vi "HELP.vi"(8 "error in (no error)":errorcluster, 11 "Instrument in":refnum<class "Instrument.lvclass">) -> (0 "error out":errorcluster, 2 "Commands":string[](array[string]), 3 "Instrument out":refnum<class "Instrument.lvclass">)   [LabVIEW 2016, in "Instrument.lvclass"]
uses:
  Instrument.lvclass
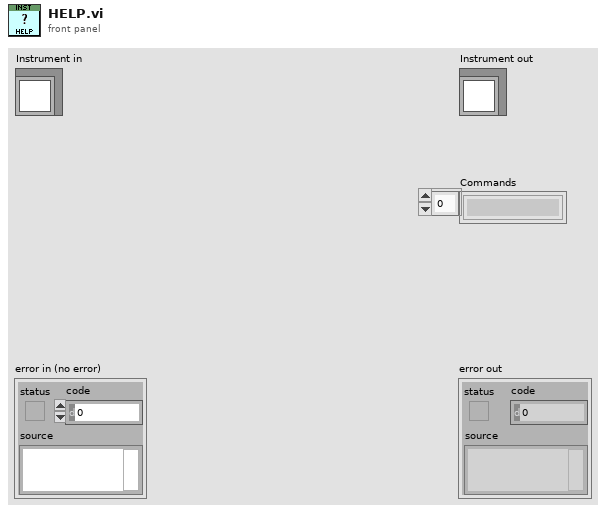
[diagram p1: front panel]
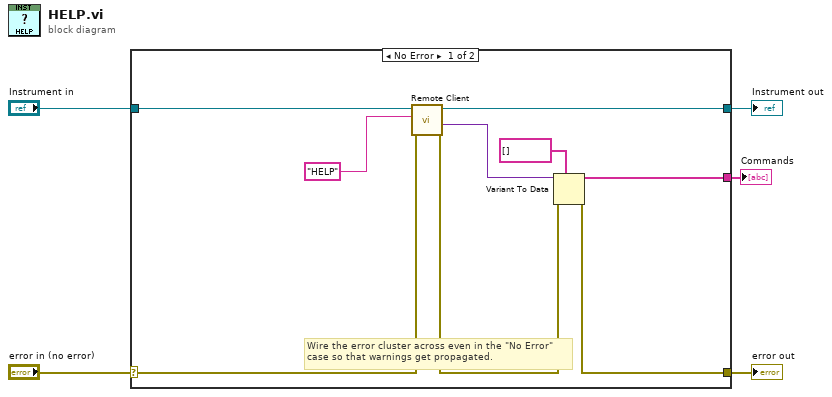
[diagram p0: block diagram]
diagram:
  n1 = case shown="No Error" "error in (no error)" {
    selector: "error in (no error)" -> [w13 w16]
    tunnel: [w8 w16] -> w4
    tunnel: [w11 w15] -> w2
    tunnel: "Instrument in" -> [w12 w15]
    tunnel: [w7 _] -> w1
    frame No Error {
      # "Wire the error cluster across even in the \"No Error\"\ncase so that warnings get propagated."
      n2 = call "Remote Client.vi"("error in (no error)"=w13, "Command"="HELP", "Instrument in"=w12) -> ("error out"=w9:errorcluster, "Data out"=w10:variant, "Instrument out"=w11:refnum<class "Instrument.lvclass">)  [unwired: 5 in, 1 out]
      n3 = Variant To Data(error in=w9, type=string[] [] ("Commands"), Variant=w10) -> (data=w7:string[], error out=w8:errorcluster)
    }
    frame Error {
    }
  }
  "error out" <- w4
  "Instrument out" <- w2
  "Commands" <- w1
